vi "Returning Values By Reference Pointer To Complex Struct.vi"(8 "error in (no error)":errorcluster, 11 "triangle":T1) -> (0 "error out":errorcluster, 2 "name":string, 3 "triangle out":T1)   [LabVIEW 2009, in "LabVIEWWrapper_PassingDataSampleDLL.lvlib"]
doc: "void ReturningValuesByReference_PointerToComplexStruct (struct complexStructPolygon* triangle);"
uses:
  <vilib>/Utility/importsl/GetValueByPointer/GetValueByPointer.xnode
  <vilib>/Utility/importsl/GetValueByPointer/datatype.ctl
  LabVIEWWrapper_PassingDataSampleDLL.lvlib
  PassingDataSampleDLL.dll
  Program Files (x86)/National Instruments/LabVIEW 2009/resource/lvimptsl.dll
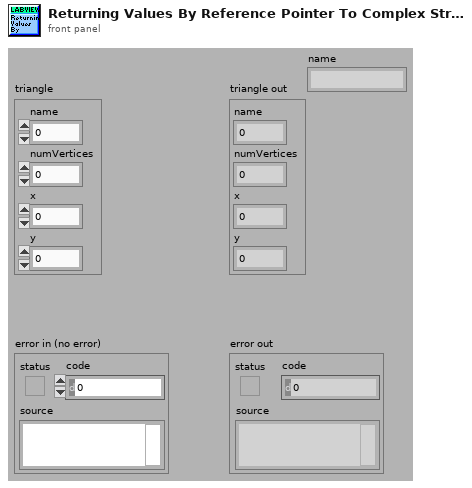
[diagram p1: front panel]
types:
  T1 = cluster{"name":u32, "numVertices":i32, "x":i32, "y":i32}
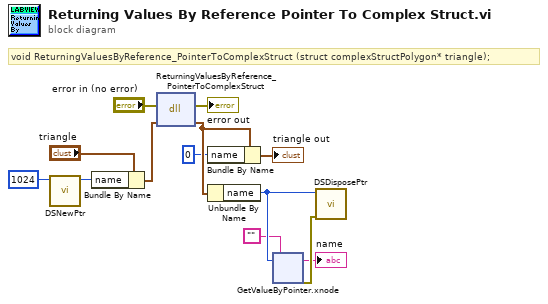
[diagram p0: block diagram]
diagram:
  # "void ReturningValuesByReference_PointerToComplexStruct (struct complexStructPolygon* triangle);"
  n1 = call <vilib>:"DSNewPtr.vi"("Size"=u64 1024) -> ("Pointer"=w11:u64)  [unwired: 9 in, 1 out]
  n2 = Bundle By Name(cluster="triangle", "name"=w11) -> (w10:T1)
  n3 = dll-call lib="C:/My Dropbox/Systems Engineering Application/SDK/C Integration/LabVIEWWrapper/PassingDataSampleDLL.*" fn="ReturningValuesByReference_PointerToComplexStruct"(error in="error in (no error)", "triangle"=w10) -> (error out=→"error out":errorcluster, "triangle"=w5:T1)  [unwired: 3 in, 1 out]
  n4 = Bundle By Name(cluster=w5, "name"=u32 0) -> (→"triangle out":T1)
  n5 = Unbundle By Name(w5) -> ("name"=w8:u32)
  n6 = xnode "GetValueByPointer.xnode"("Pointer"=w8, "InputType"="") -> ("Output"=→"name":string, "ErrorOut"=w9:errorcluster)  [unwired: 2 in]
  n7 = call <vilib>:"DSDisposePtr.vi"("error in (no error)"=w9, "Pointer"=w8) -> ()  [unwired: 9 in, 1 out]
